vi "multiplex.vi"(9 "in 3":bool, 10 "in 2":bool, 11 "in 1":bool) -> (1 "out 3":bool, 2 "out 2":bool, 3 "out 1":bool)   [LabVIEW 2012]
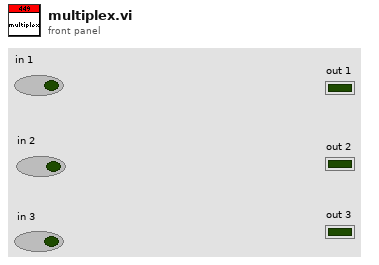
[diagram p1: front panel]
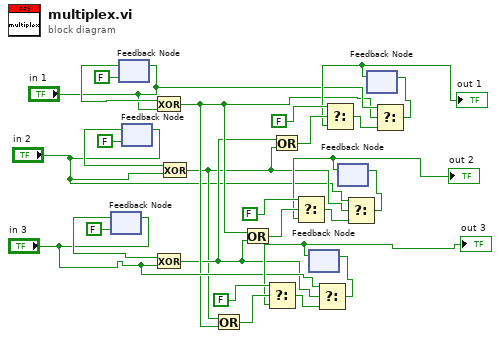
[diagram p0: block diagram]
diagram:
  n1 = feedback #1(FALSE ("in 1")) -> (w22:bool)
  n2 = feedback-in #1("in 3") -> ()
  n3 = feedback #2(FALSE ("in 1")) -> (w24:bool)
  n4 = feedback-in #2("in 1") -> ()
  n5 = feedback #3(FALSE ("in 1")) -> (w23:bool)
  n6 = feedback-in #3("in 2") -> ()
  n7 = Exclusive Or(1:"in 1", 2:w24) -> (0:w4:bool)
  n8 = Exclusive Or(1:"in 3", 2:w22) -> (0:w3:bool)
  n9 = Exclusive Or(1:"in 2", 2:w23) -> (0:w2:bool)
  n10 = Or(x=w2, y=w4) -> (x .or. y?=w12:bool)
  n11 = Or(x=w4, y=w3) -> (x .or. y?=w16:bool)
  n12 = Or(x=w3, y=w2) -> (x .or. y?=w21:bool)
  n13 = feedback #4() -> (w8:bool)  [unwired: 1 in]
  "out 3" <- w8
  n14 = Select(t=FALSE, s=w12, f=w8) -> (s? t:f=w9:bool)
  n15 = Select(t="in 3", s=w3, f=w9) -> (s? t:f=w10:bool)
  n16 = feedback-in #4(w10) -> ()
  n17 = feedback #5() -> (w7:bool)  [unwired: 1 in]
  "out 2" <- w7
  n18 = Select(t=FALSE, s=w16, f=w7) -> (s? t:f=w13:bool)
  n19 = Select(t="in 2", s=w2, f=w13) -> (s? t:f=w14:bool)
  n20 = feedback-in #5(w14) -> ()
  n21 = feedback #6() -> (w19:bool)  [unwired: 1 in]
  "out 1" <- w19
  n22 = Select(t=FALSE, s=w21, f=w19) -> (s? t:f=w17:bool)
  n23 = Select(t="in 1", s=w4, f=w17) -> (s? t:f=w18:bool)
  n24 = feedback-in #6(w18) -> ()
